vi "RemoveKey.vi"(8 "键":string="d", 11 "键值串":string="[a=a][b=b][c=c]") -> (0 "删除的值":string, 3 "删除后的键值串":string="[a=a][b=b][c=c]")   [LabVIEW 2020, in "Curve Editor.lvlib" / "Key Value.lvlib"]
uses:
  Key Value.lvlib
panel:
  out "存在?":bool
  # "从键值串中删除键，并返回删除后的键值串及被删除的键的值"
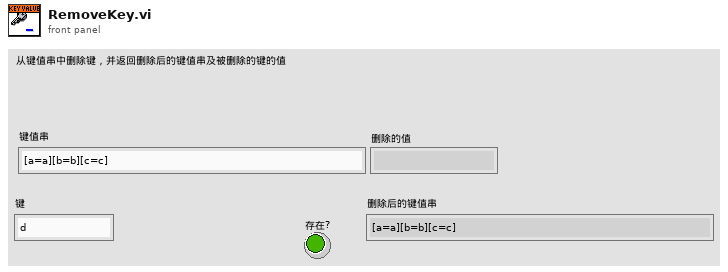
[diagram p1: front panel]
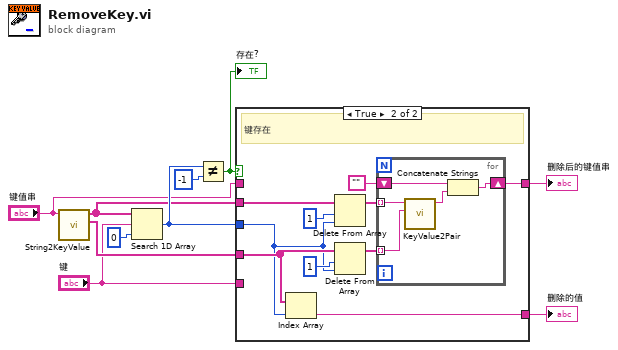
[diagram p0: block diagram]
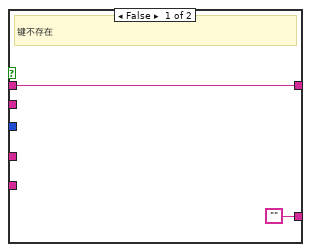
[diagram p2: hidden frame]
diagram:
  n1 = call "String2KeyValue.vi"("健值对字符串"="键值串") -> ("值数组"=w7:string[], "键数组"=w1:string[])  [unwired: 9 in]
  n2 = Search 1D Array(1D array=w1, element="键", start index (0)=0 ("开始索引(0)")) -> (index of element=w6:i32)
  n3 = Not Equal?(x=w6, y=-1) -> (x != y?=w8:bool)
  "存在?" <- w8
  n4 = case shown="True" w8 {
    tunnel: w7 -> [_ w21]
    tunnel: w6 -> [_ w17]
    tunnel: "键" -> [_ _]
    tunnel: ["" w22] -> w4
    tunnel: "键值串" -> [w11 _]
    tunnel: [w11 w13] -> w2
    tunnel: w1 -> [_ w20]
    frame False {
      # "键不存在"
    }
    frame True {
      # "键存在"
      n5 = Index Array(array=w21, index=w17) -> (element=w22:string)
      n6 = Delete From Array(array=w20, length=1 ("长度"), index=w17) -> (array with subset deleted=w16:string[])  [unwired: 1 out]
      n7 = Delete From Array(array=w21, length=1 ("长度"), index=w17) -> (array with subset deleted=w15:string[])  [unwired: 1 out]
      n8 = for {
        tunnel: w16 -> [w27] mode=indexing
        tunnel: w15 -> [w26] mode=indexing
        shift-right: [w24] -> w13
        shift-left: "" -> [w23]
        n9 = call "KeyValue2Pair.vi"("值"=w26, "键"=w27) -> ("键值对"=w25:string)  [unwired: 9 in]
        n10 = Concatenate Strings(w23, w25) -> (w24:string)
      }
    }
  }
  "删除的值" <- w4
  "删除后的键值串" <- w2
